vi "Compare_IsSame_NoUI.vi"() -> ()   [LabVIEW 2022 SP3]
panel:
  out "error out":errorcluster
  out "Same?":bool
  in  "Current VI":path
  # "Run thi vi from the project C:\\Users\\inigo\\Documents\\Kbiosystems\\LabVIEW Utilities\\compare VIs.lvproj\nrunnign outside the project does not launch the labview compare tool in interactive mode"
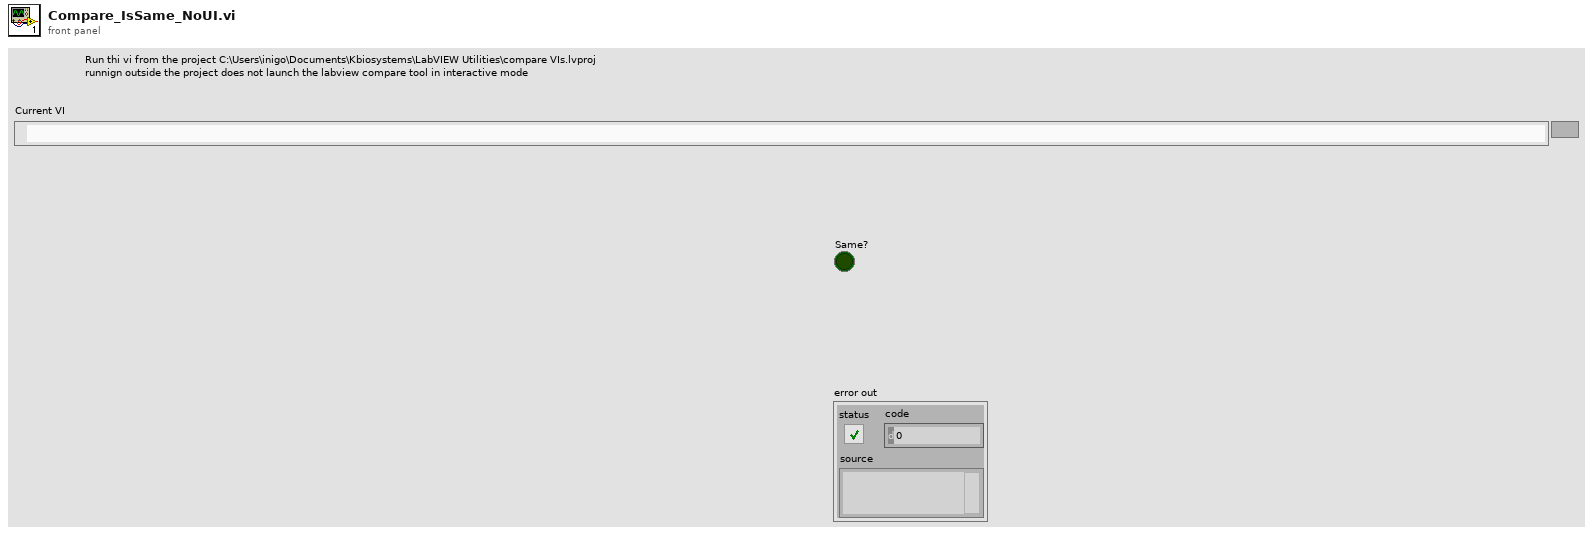
[diagram p1: front panel]
types:
  T1 = enum16{"Left Button", "Center Button", "Right Button", "Window Close"}
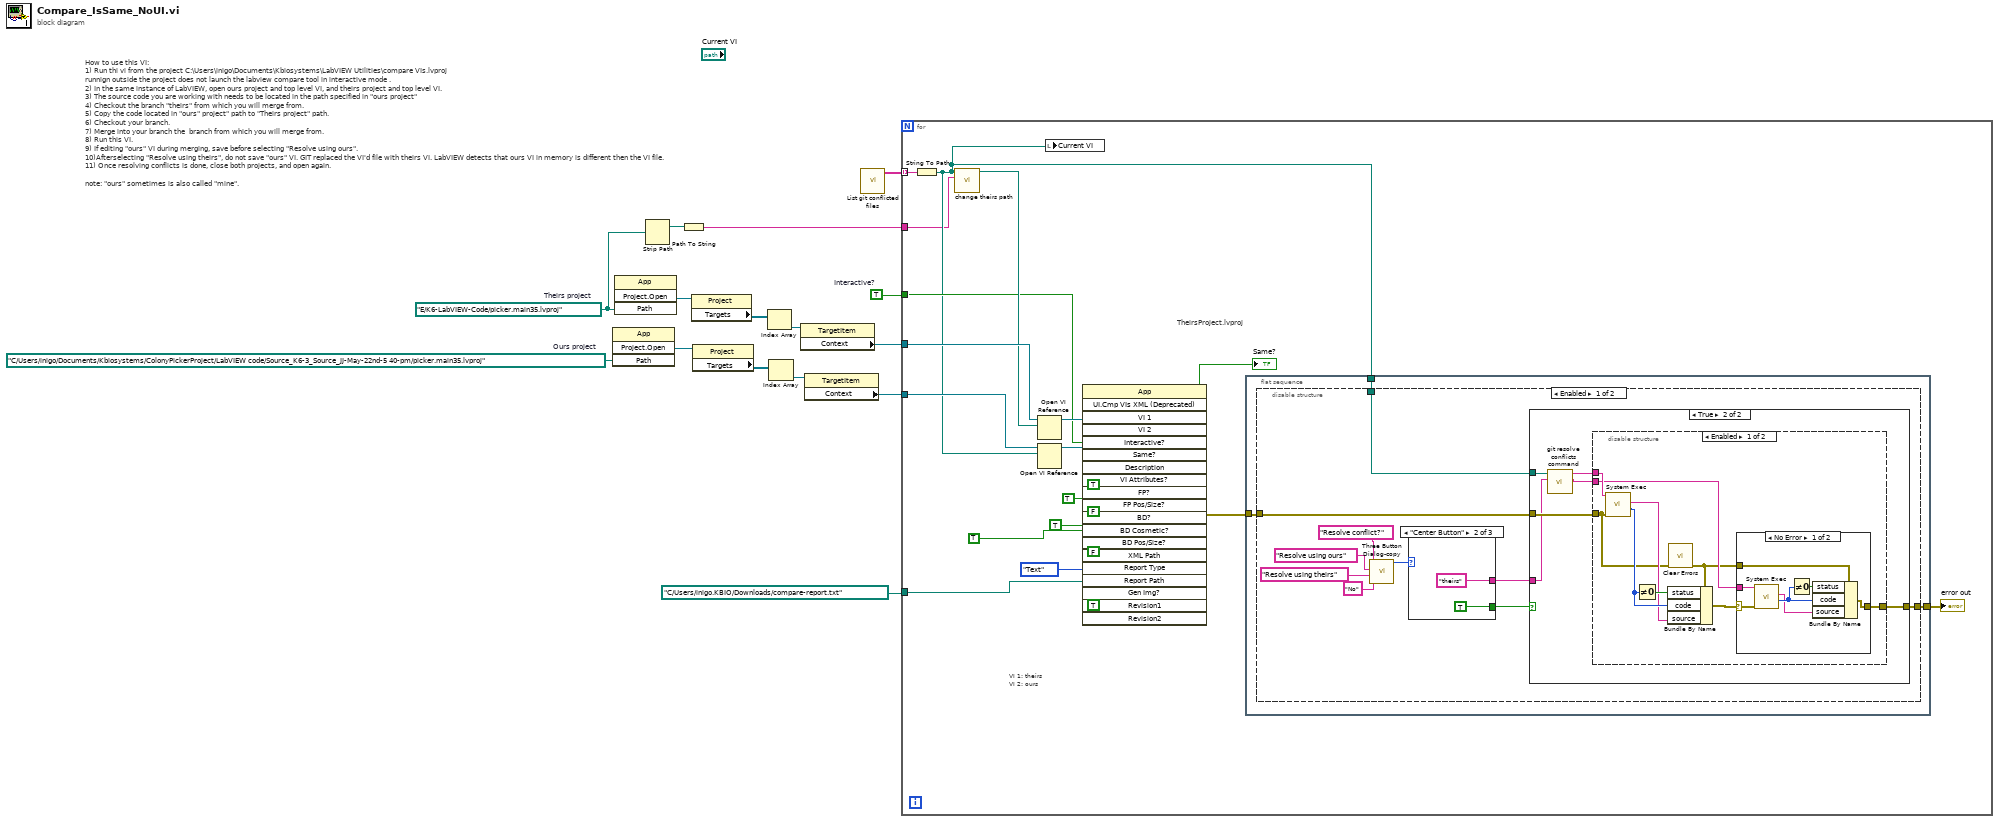
[diagram p0: block diagram]
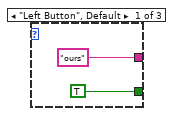
[diagram p2: hidden frame]
diagram:
  w4 = TRUE  # Interactive?
  w15 = path "C:/Users/inigo/Documents/Kbiosystems/ColonyPickerProject/LabVIEW code/Source_K6-3_Source_JJ-May-22nd-5 40-pm/picker.main35.lvproj"  # Ours project
  w3 = path "E:/K6-LabVIEW-Code/picker.main35.lvproj"  # Theirs project
  # "How to use this VI:\n1) Run thi vi from the project C:\\Users\\inigo\\Documents\\Kbiosystems\\LabVIEW Utilities\\compare VIs.lvproj\nrunnign outside the project does not launch the labview compare tool in interactive mode .\n2) In the same instance of LabVIEW, open ours project and top level VI, and theirs project and top level VI.\n3) The source code you are working with needs to be located in the path specified in \"ours project\"\n4) Checkout the branch \"theirs\" from which you will merge from.\n5) Copy the code located in \"ours\" project\" path to \"Theirs project\" path.\n6) Checkout your branch.\n7) Merge into your branch the  branch from which you will merge from.\n8) Run this VI.\n9) If editing \"ours\" VI during merging, save before selecting \"Resolve using ours\".\n10)Afterselecting \"Resolve using theirs\", do not save \"ours\" VI. GIT replaced the VI'd file with theirs VI. LabVIEW detects that ours VI in memory is different then the VI file. \n11) Once resolving conflicts is done, close both projects, and open again. \n\nnote: \"ours\" sometimes is also called \"mine\"."
  n1 = invoke class="App" method="Project.Open"("Path"=w15) -> ("Project:Open"=w11:refnum<vi>)  [unwired: 3 in, 3 out]
  n2 = invoke class="App" method="Project.Open"("Path"=w3) -> ("Project:Open"=w14:refnum<vi>)  [unwired: 3 in, 3 out]
  n3 = Strip Path(path=w3) -> (stripped path=w2:path)  [unwired: 1 out]
  n4 = Path To String(path=w2) -> (string=w1:string)
  n5 = property class="Project"(reference=w14) -> ("Targets"=w13:refnum<vi>[])  [unwired: 1 in, 2 out]
  n6 = property class="Project"(reference=w11) -> ("Targets"=w12:refnum<vi>[])  [unwired: 1 in, 2 out]
  n7 = Index Array(array=w13) -> (element=w10:refnum<vi>)  [unwired: 1 in]
  n8 = Index Array(array=w12) -> (element=w9:refnum<vi>)  [unwired: 1 in]
  n9 = property class="TargetItem"(reference=w10) -> ("Context"=w8:refnum<vi>)  [unwired: 1 in, 2 out]
  n10 = property class="TargetItem"(reference=w9) -> ("Context"=w7:refnum<vi>)  [unwired: 1 in, 2 out]
  n11 = call "List git conflicted files.vi"() -> ("conflicted files list"=w6:string[])  [unwired: 10 in, 1 out]
  n12 = for {
    tunnel: w8 -> [w30]
    tunnel: w7 -> [w29]
    tunnel: w6 -> [w20] mode=indexing
    tunnel: w4 -> [w19]
    tunnel: path "C:/Users/inigo.KBIO/Downloads/compare-report.txt" ("Result JSON Path") -> [w18]
    tunnel: w1 -> [w16]
    # "VI 1: theirs\nVI 2: ours"
    # "TheirsProject.lvproj"
    n13 = String To Path(string=w20) -> (path=w17:path)
    n14 = call "change theirs path.vi"("theirs path"=w16, "Path in"=w17) -> ("path out"=w24:path)  [unwired: 9 in]
    n15 = Open VI Reference(application reference (local)=w30, vi path=w24) -> (vi reference=w35:refnum<vi>)  [unwired: 4 in, 1 out]
    n16 = Open VI Reference(application reference (local)=w29, vi path=w17) -> (vi reference=w34:refnum<vi>)  [unwired: 4 in, 1 out]
    n17 = local write "Current VI"(w17) -> ()
    n18 = invoke class="App" method="UI.Cmp VIs XML (Deprecated)"("VI 1"=w35, "VI 2"=w34, "Interactive?"=w19, "VI Attributes?"=TRUE, "FP?"=TRUE, "FP Pos/Size?"=FALSE, "BD?"=TRUE, "BD Cosmetic?"=TRUE, "BD Pos/Size?"=FALSE, "Report Type"=enum32{"None", "Webpage", "Text", "MS Word"}."Text", "Report Path"=w18, "Gen Img?"=TRUE) -> (error out=w23:errorcluster, "Same?"=→"Same?":bool)  [unwired: 8 in, 18 out]
    n19 = flat-sequence {
      tunnel: w23 -> [w39]
      tunnel: [w38] -> w36
      tunnel: w17 -> [w37]
      frame #0 {
        n20 = disable-structure shown="Enabled" {
          disable-tunnel: w39 -> [w49 w79]
          disable-tunnel: [w48 w79] -> w38
          disable-tunnel: w37 -> [w47 _]
          frame Enabled {
            n21 = call "Three Button Dialog-copy.vi"("Right Button Text (\"Cancel\")"="No" ("Right Button Text (\"Cancel\")"), "Center Button Text (\"No\")"="Resolve using theirs" ("Center Button Text (\"No\")"), "Left Button Text (\"Yes\")"="Resolve using ours" ("Left Button Text (\"Yes\")"), "message"="Resolve conflict?") -> ("Which Button?"=w46:T1)  [unwired: 7 in]
            n22 = case shown="\"Center Button\"" w46 {
              tunnel: ["ours" "theirs" _] -> w40
              tunnel: [TRUE TRUE _] -> w41
              frame "Left Button", Default {
              }
              frame "Center Button" {
              }
              frame "Right Button" {
              }
            }
            n23 = case shown="True" w41 {
              tunnel: w49 -> [w54 w60]
              tunnel: [w54 w59] -> w48
              tunnel: w47 -> [_ w57]
              tunnel: w40 -> [_ w56]
              frame False {
              }
              frame True {
                n24 = call "git resolve conflicts command.vi"("Choosen file"=w56, "ours vi path"=w57) -> ("git stage file"=w55:string, "git resolve conficts cmd"=w58:string)  [unwired: 8 in]
                n25 = disable-structure shown="Enabled" {
                  disable-tunnel: w60 -> [w65 w78]
                  disable-tunnel: [w62 w78] -> w59
                  disable-tunnel: w58 -> [w66 _]
                  disable-tunnel: w55 -> [w63 _]
                  frame Enabled {
                    n26 = call <vilib>:"System Exec.vi"("error in (no error)"=w65, "command line"=w66) -> ("return code"=w68:i32, "standard error"=w67:string)  [unwired: 6 in, 2 out]
                    n27 = Not Equal To 0?(x=w68) -> (x != 0?=w69:bool)
                    n28 = call <vilib>:"Clear Errors.vi"("error in (no error)"=w65) -> ("error out"=w61:errorcluster)  [unwired: 5 in, 1 out]
                    n29 = Bundle By Name(cluster=w61, "status"=w69, "code"=w68, "source"=w67) -> (w64:errorcluster)
                    n30 = case shown="No Error" w64 {
                      selector: w64 -> [w76 w77]
                      tunnel: w63 -> [w75 _]
                      tunnel: [w70 w77] -> w62
                      tunnel: w61 -> [w71 _]
                      frame No Error {
                        n31 = call <vilib>:"System Exec.vi"("error in (no error)"=w76, "command line"=w75) -> ("return code"=w74:i32, "standard error"=w72:string)  [unwired: 6 in, 2 out]
                        n32 = Not Equal To 0?(x=w74) -> (x != 0?=w73:bool)
                        n33 = Bundle By Name(cluster=w71, "status"=w73, "code"=w74, "source"=w72) -> (w70:errorcluster)
                      }
                      frame Error {
                      }
                    }
                  }
                  frame Disabled {
                  }
                }
              }
            }
          }
          frame Disabled {
          }
        }
      }
    }
    "error out" <- w36
  }
